vi "Write WebSocket Connection.vi"(8 "error in (no error)":errorcluster, 10 "WebSocket Connection":refnum<k5>, 11 "WebSocket Connection in":refnum<class "WebSocket Connection.lvclass">) -> (0 "error out":errorcluster, 3 "WebSocket Connection out":refnum<class "WebSocket Connection.lvclass">)   [LabVIEW 2016, in "WebSocket Actors.lvlib" / "WebSocket Connection.lvclass"]
uses:
  WebSocket Connection.lvclass
  WebSocket Connection.lvclass/WebSocket Connection.ctl
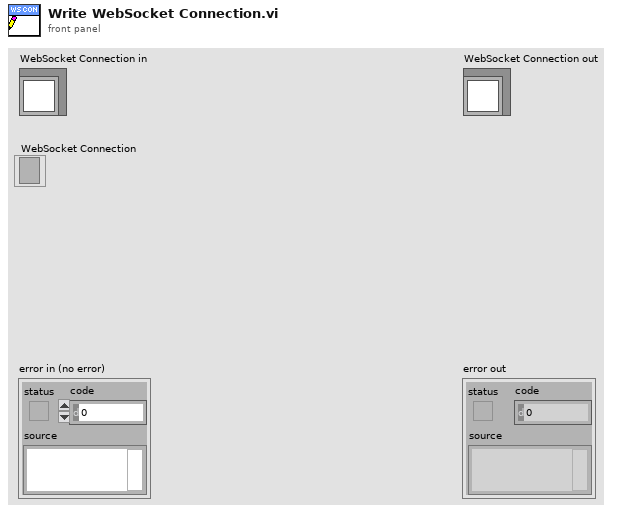
[diagram p1: front panel]
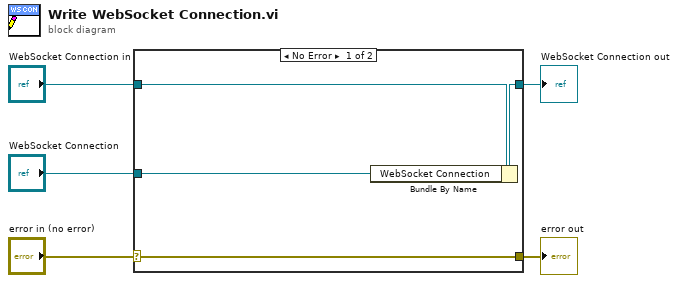
[diagram p0: block diagram]
diagram:
  n1 = case shown="No Error" "error in (no error)" {
    selector: "error in (no error)" -> [w9 w10]
    tunnel: [w9 w10] -> w4
    tunnel: [w7 w11] -> w2
    tunnel: "WebSocket Connection in" -> [w8 w11]
    tunnel: "WebSocket Connection" -> [w6 _]
    frame No Error {
      n2 = Bundle By Name(cluster=w8, "WebSocket Connection"=w6) -> (w7:refnum<class "WebSocket Connection.lvclass">)
    }
    frame Error {
    }
  }
  "error out" <- w4
  "WebSocket Connection out" <- w2
